vi "Transcriptor LabVIEW to C code Step 3 Translate Elements.vi"(8 "error in (no error)":errorcluster, 11 "Diagram in":refnum<vi>) -> (0 "error out":errorcluster, 1 "transcripted C code":string[](array[string]), 2 "feedback and other output assignments":string[](array[string]), 3 "transcriptor cluster":T1[](array[typedef]))   [LabVIEW 2014]
uses:
  types/LabVIEW Universal Transcriptor Cluster.ctl
  <vilib>/Utility/miscctls.llb/LVPointTypeDef.ctl
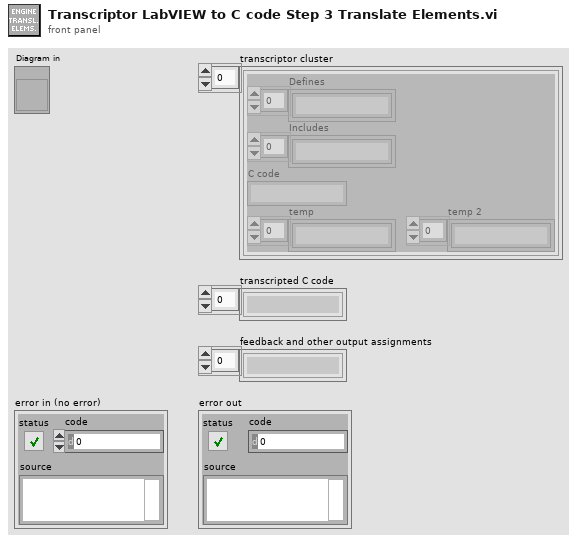
[diagram p1: front panel]
types:
  T1 = typedef "LabVIEW Universal Transcriptor Cluster.ctl" = cluster{"Defines":string[], "Includes":string[], "C code":string, "temp":string[], "temp 2":string[]}
  T2 = typedef "LVPointTypeDef.ctl" = cluster{"Horizontal":i16, "Vertical":i16}
  T3 = cluster{"wire labels":string[], "wire terminals datatypes":string[][]}
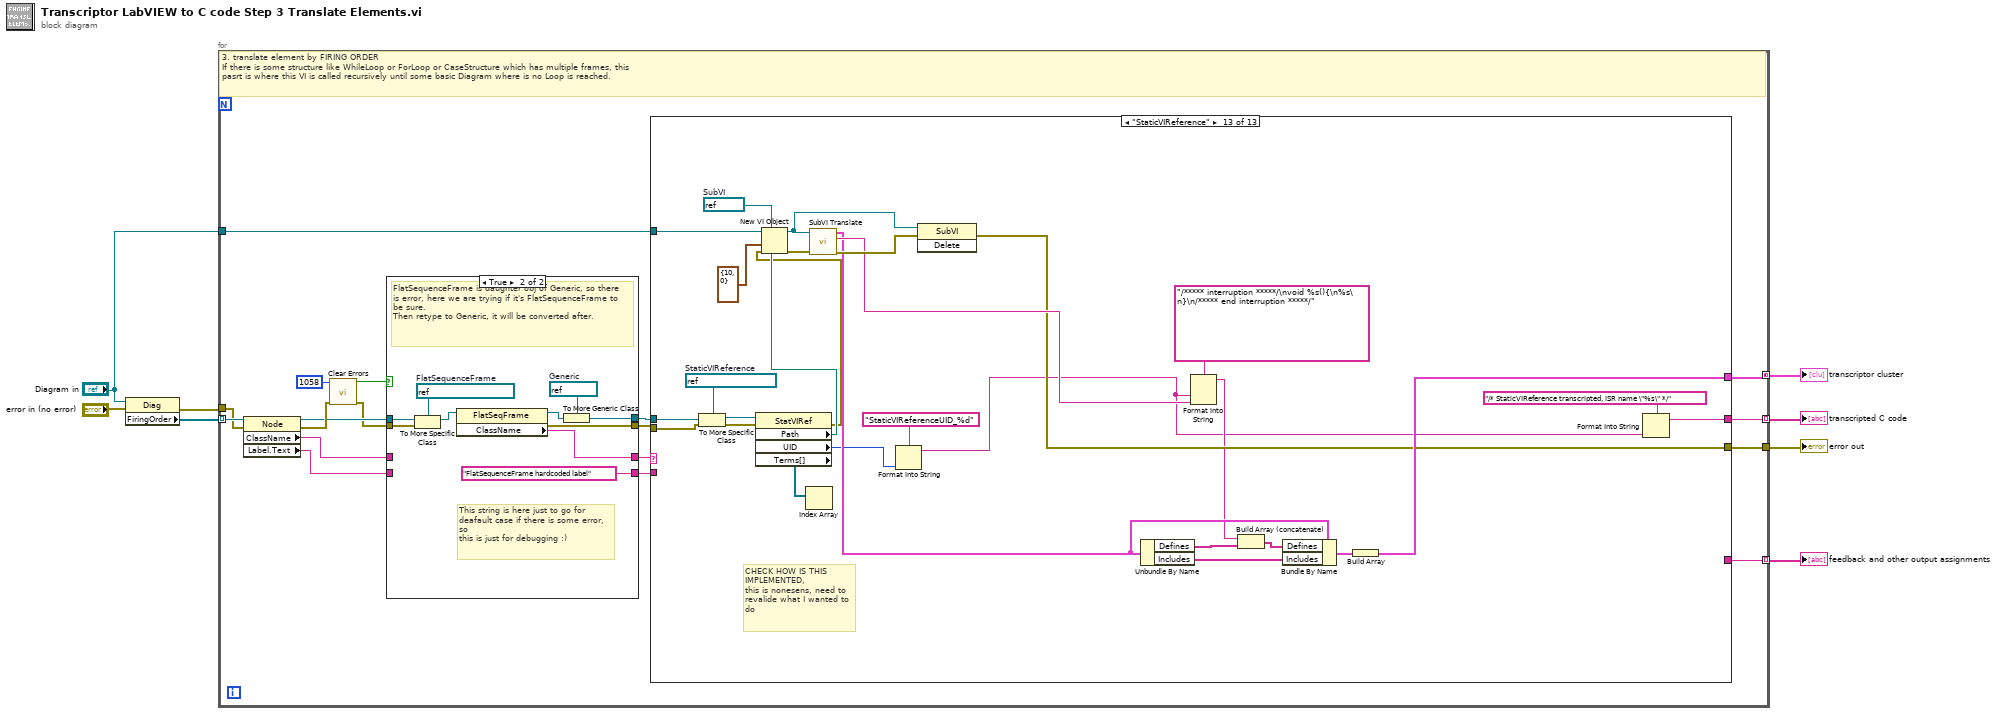
[diagram p0: block diagram]
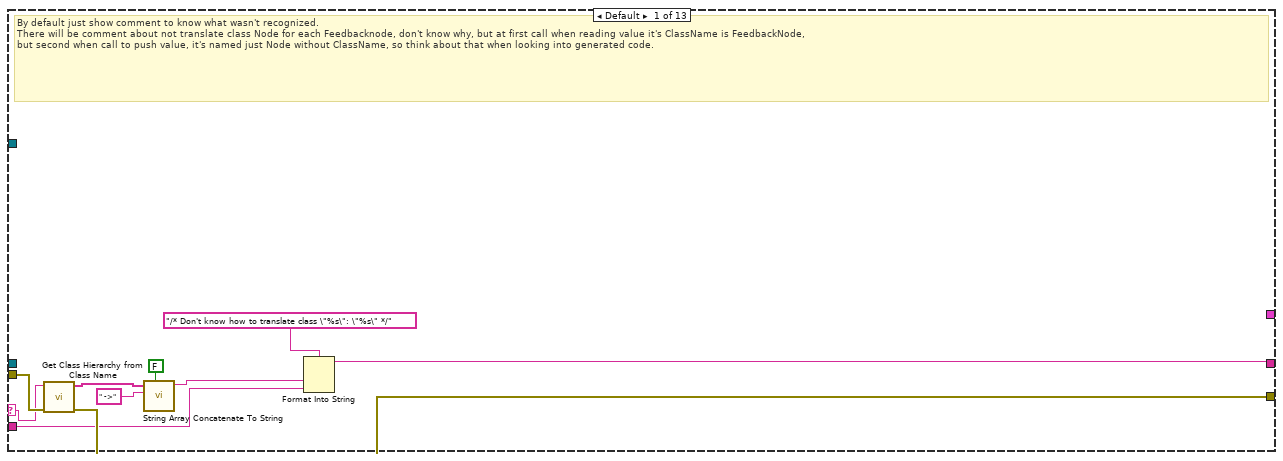
[diagram p3: hidden frame]
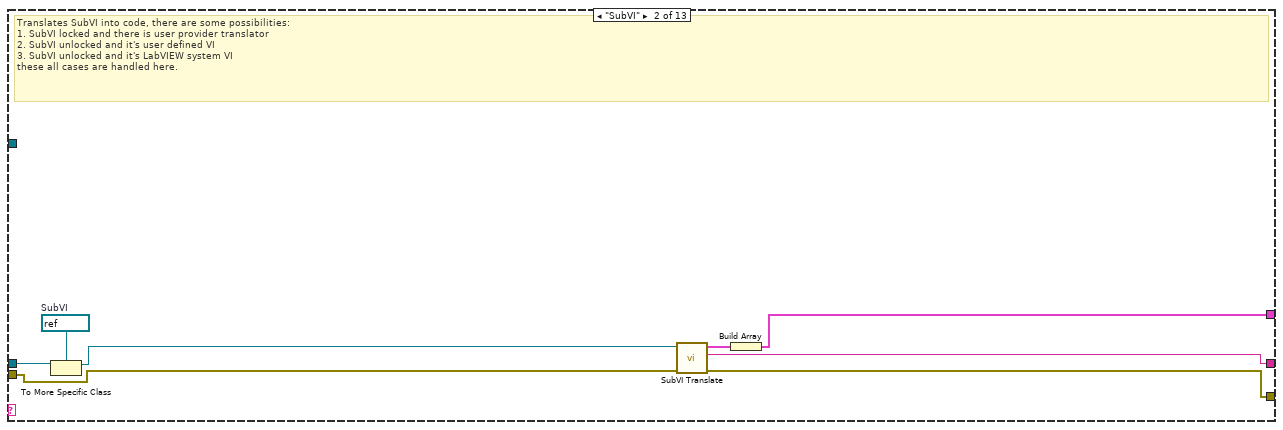
[diagram p4: hidden frame]
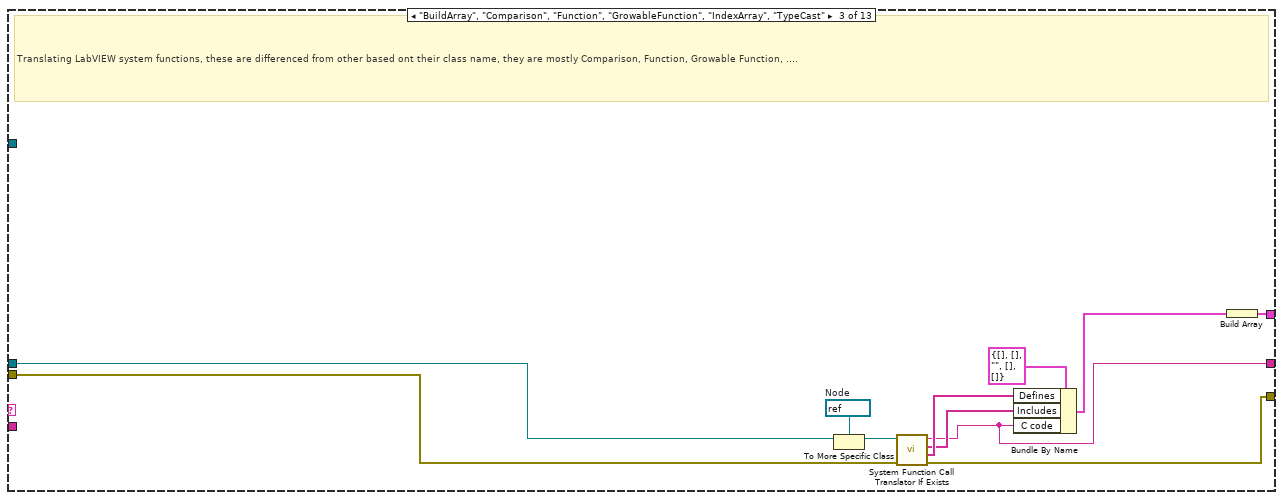
[diagram p5: hidden frame]
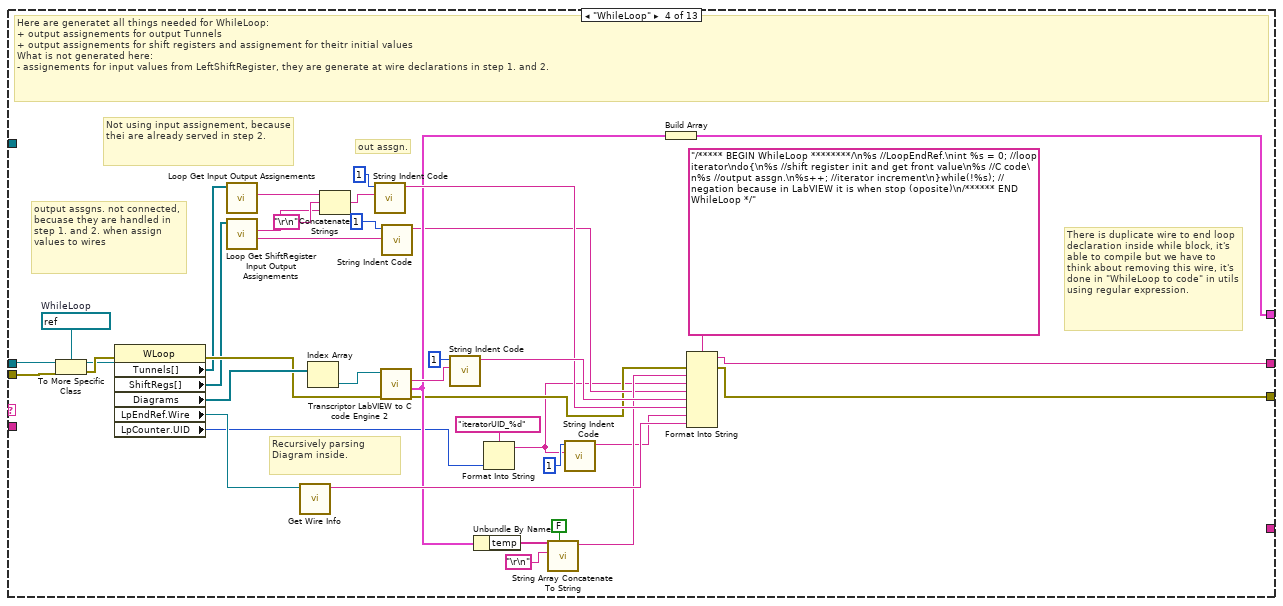
[diagram p6: hidden frame]
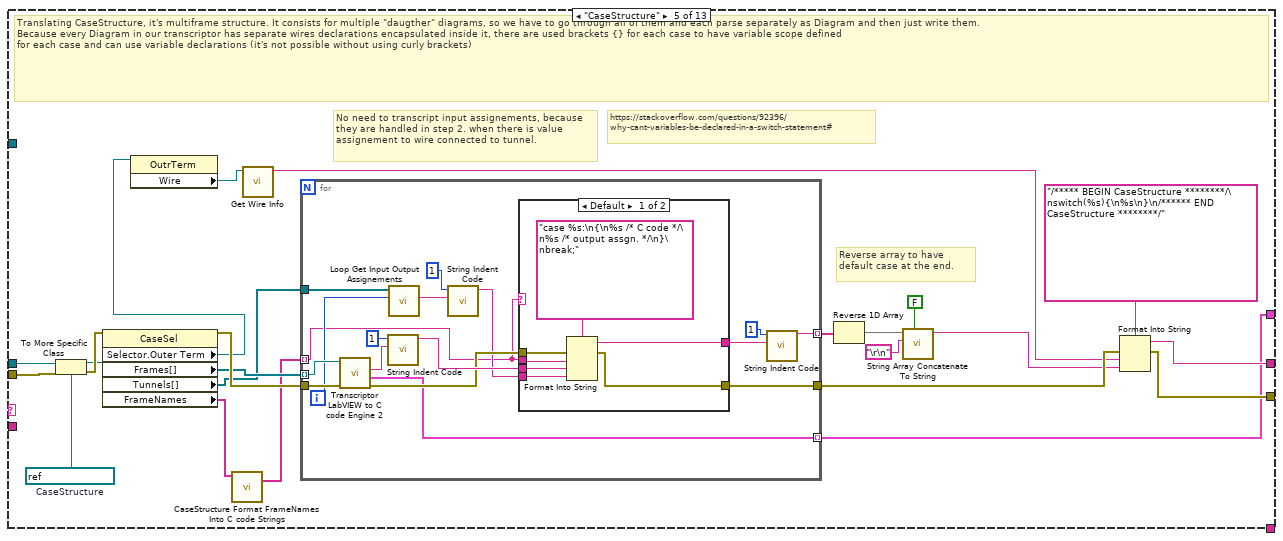
[diagram p7: hidden frame]
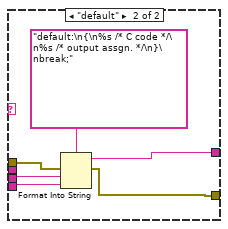
[diagram p8: hidden frame]
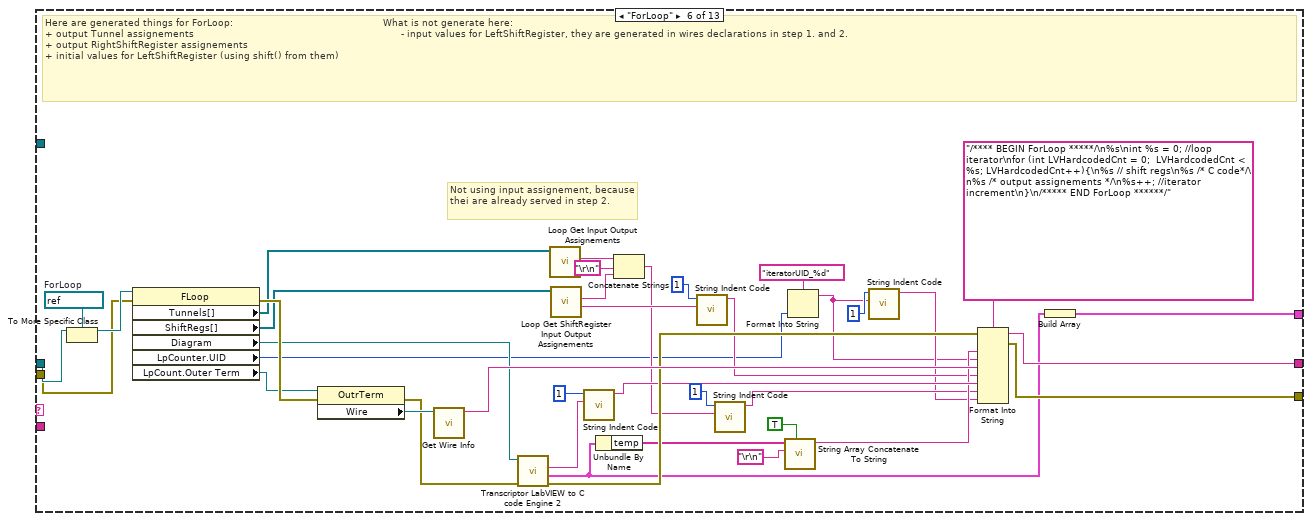
[diagram p9: hidden frame]
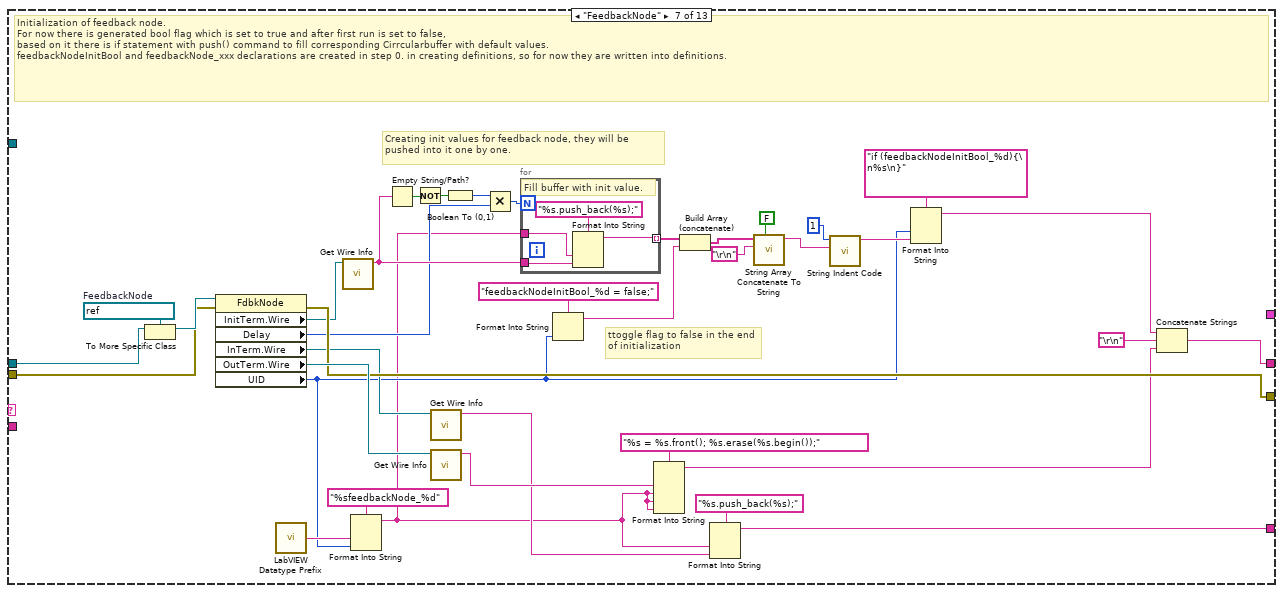
[diagram p10: hidden frame]
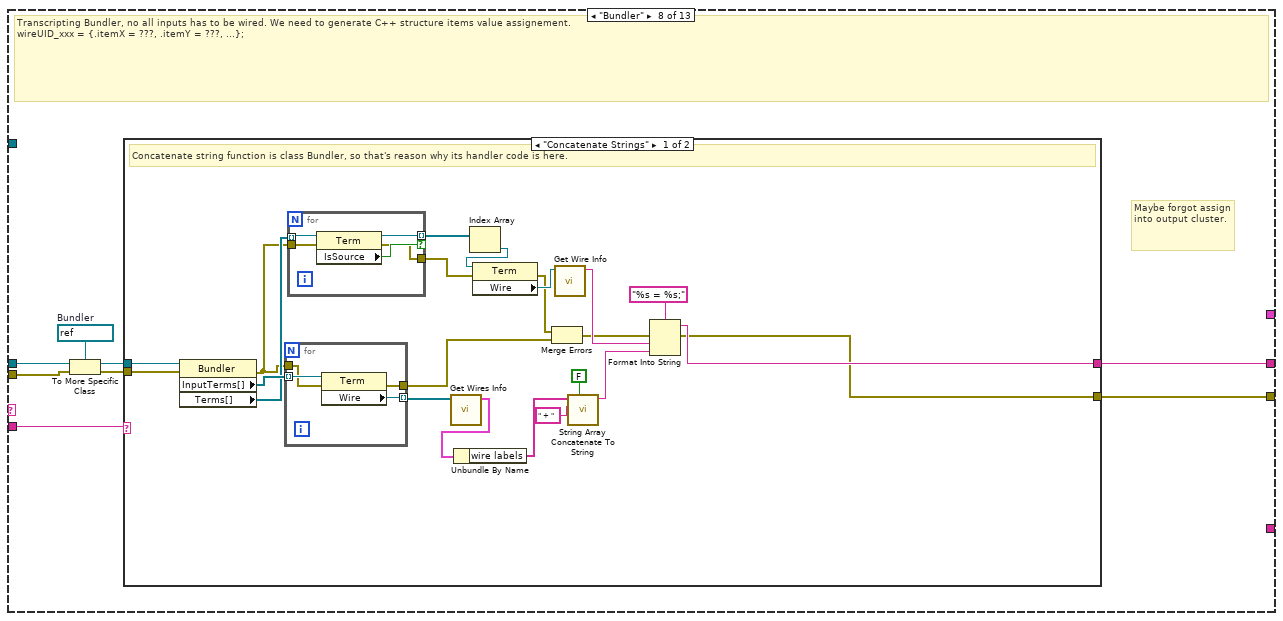
[diagram p11: hidden frame]
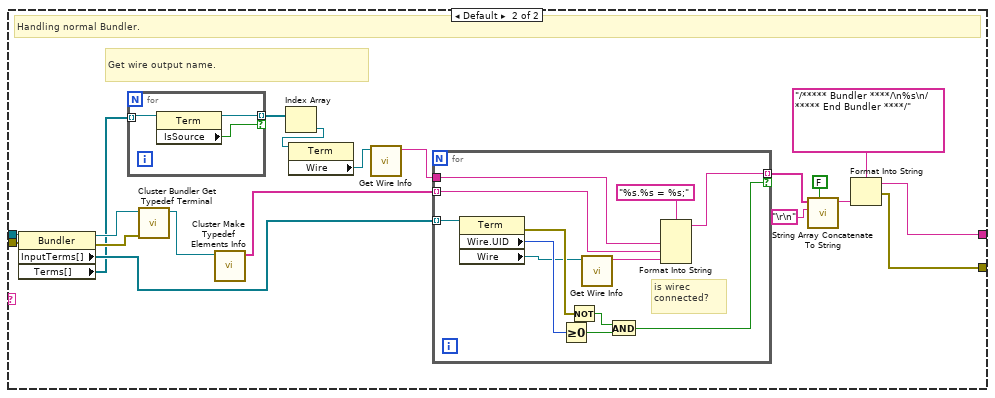
[diagram p12: hidden frame]
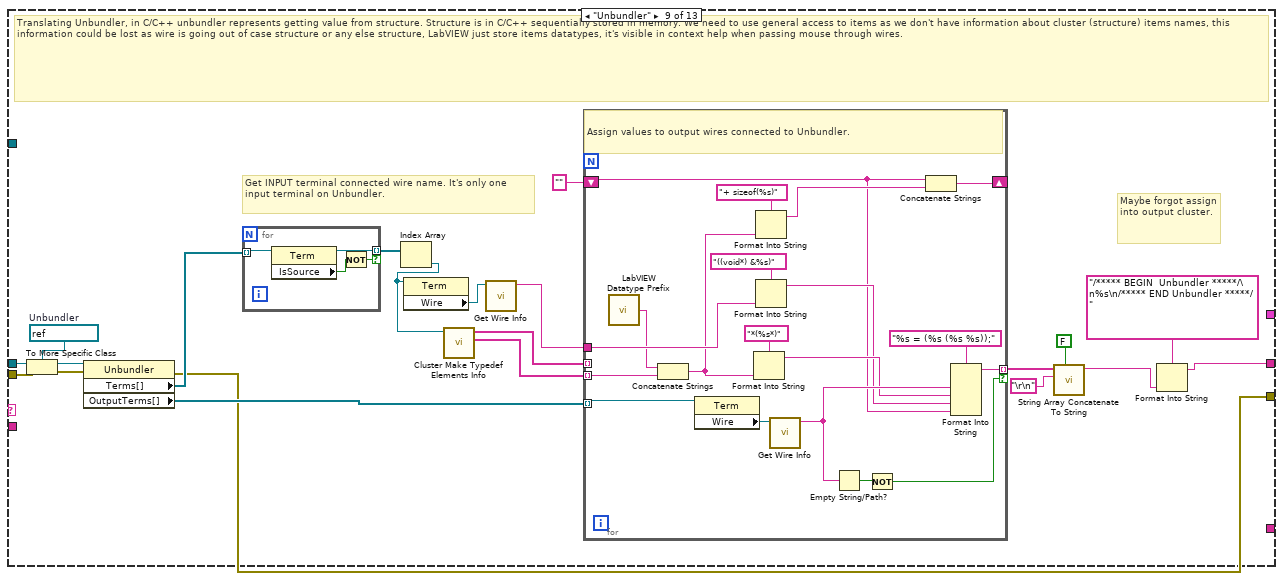
[diagram p13: hidden frame]
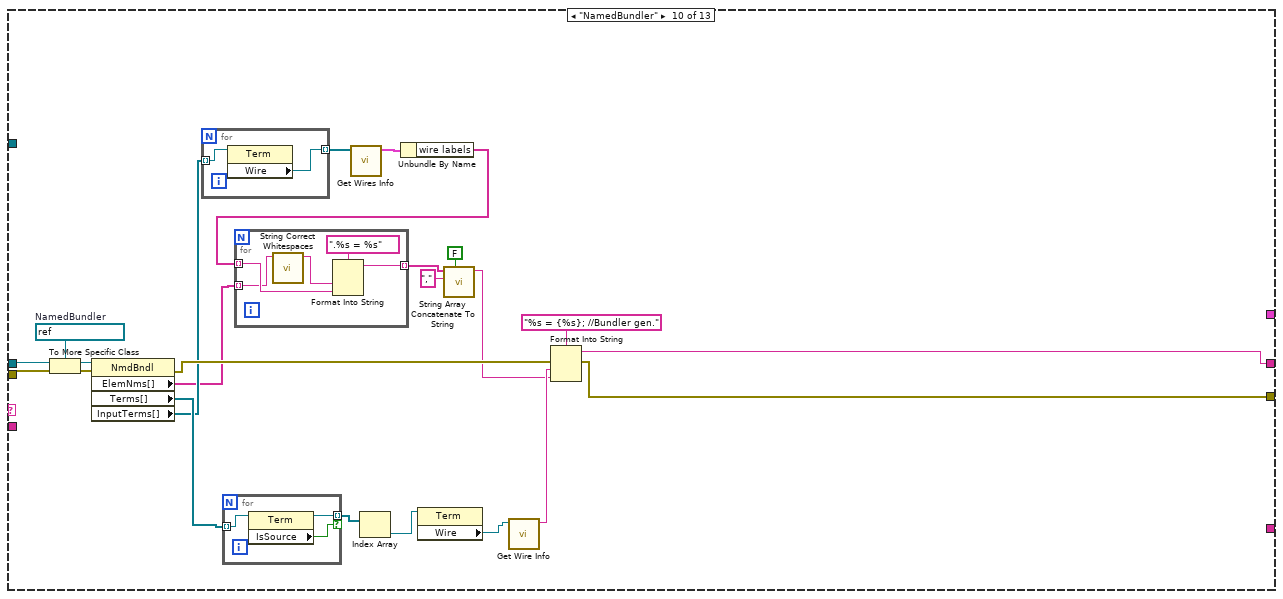
[diagram p14: hidden frame]
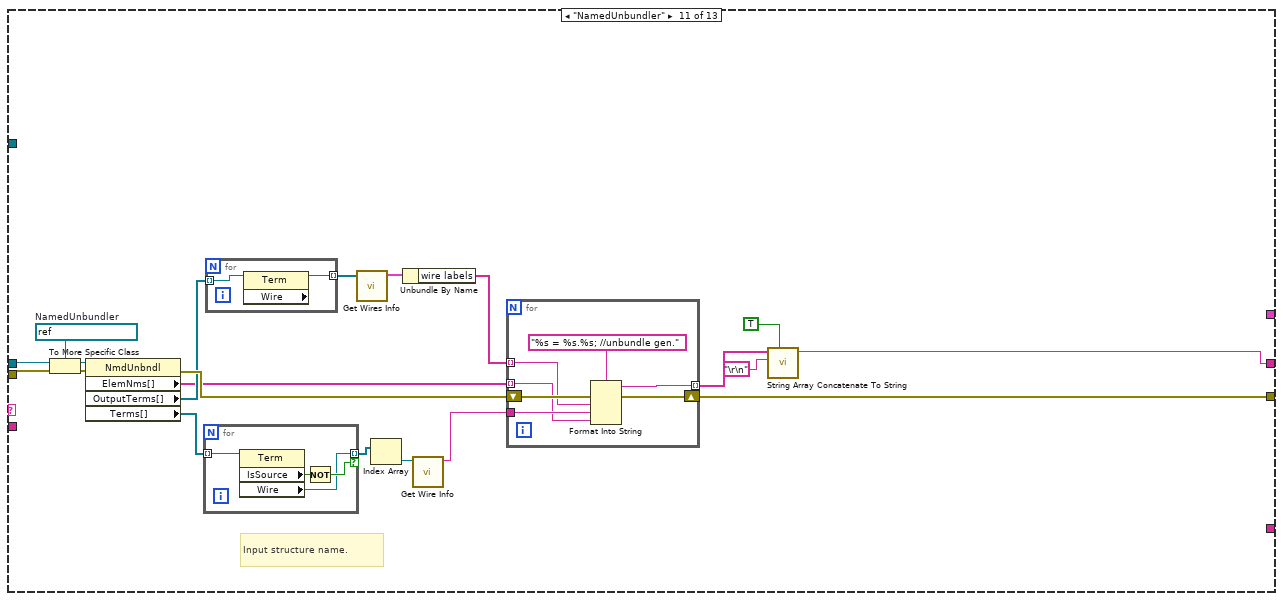
[diagram p15: hidden frame]
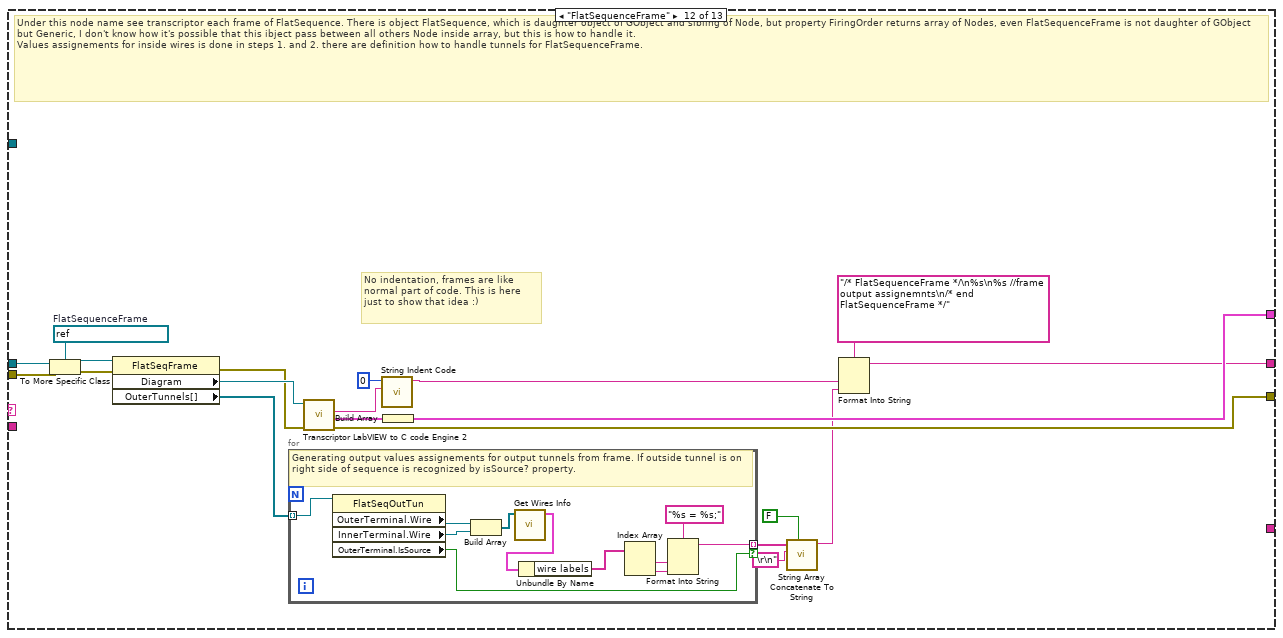
[diagram p16: hidden frame]
diagram:
  n1 = property on="Property Node" class="Diag"(reference="Diagram in", error in="error in (no error)") -> (error out=w3:errorcluster, "FiringOrder"=w8:refnum<vi>[])  [unwired: 1 out]
  n2 = for {
    tunnel: w8 -> [w26] mode=indexing
    tunnel: w3 -> [w25]
    tunnel: [w22] -> w4 mode=indexing
    tunnel: [w21] -> w6
    tunnel: [w24] -> w2 mode=concatenating
    tunnel: [w23] -> w7 mode=indexing
    tunnel: "Diagram in" -> [w9]
    # "3. translate element by FIRING ORDER\nIf there is some structure like WhileLoop or ForLoop or CaseStructure which has multiple frames, this\npasrt is where this VI is called recursively until some basic Diagram where is no Loop is reached."
    n3 = property class="Node"(reference=w26, error in=w25) -> (reference out=w18:refnum<vi>, error out=w20:errorcluster, "ClassName"=w13:string, "Label.Text"=w12:string)
    n4 = call <vilib>:"Clear Errors.vi"("error in (no error)"=w20, "specific error code to clear (0: all)"=1058) -> ("error out"=w17:errorcluster, "specific error cleared?"=w16:bool)  [unwired: 4 in]
    n5 = case shown="True" w16 {
      tunnel: w18 -> [w27 w40]
      tunnel: w17 -> [w28 w39]
      tunnel: [w30 w36] -> w15
      tunnel: [w29 "FlatSequenceFrame hardcoded label" ("Label.Text")] -> w14
      tunnel: w13 -> [w30 _]
      tunnel: w12 -> [w29 _]
      tunnel: [w28 w35] -> w11
      tunnel: [w27 w31] -> w10
      frame False {
        # "No error, so we are parsing some Node."
      }
      frame True {
        w33 = refnum<vi> refnum  # Generic
        w38 = refnum<vi> refnum  # FlatSequenceFrame
        # "This string is here just to go for\ndeafault case if there is some error, so\nthis is just for debugging :)"
        # "FlatSequenceFrame is daughter obj of Generic, so there is error, here we are trying if it's FlatSequenceFrame to be sure.\nThen retype to Generic, it will be converted after."
        n6 = To More Specific Class(target class=w38, reference=w40, error in=w39) -> (specific class reference=w37:refnum<vi>)  [unwired: 1 out]
        n7 = property class="FlatSeqFrame"(reference=w37) -> (reference out=w32:refnum<vi>, error out=w35:errorcluster, "ClassName"=w36:string)  [unwired: 1 in]
        n8 = To More Generic Class(target class=w33, reference=w32) -> (generic class reference=w31:refnum<vi>)
      }
    }
    n9 = case shown="\"StaticVIReference\"" w15 {
      selector: w15 -> [w41 _ _ _ _ _ _ _ _ _ _ _ _]
      tunnel: w10 -> [_ w58 w61 w108 w114 w200 w237 w248 w332 w381 w411 w444 w483]
      tunnel: [w49 w55 w66 w100 w126 w190 w210 w243 w315 w368 w392 w430 w460] -> w22
      tunnel: w11 -> [w44 w54 w69 w104 w129 w197 w229 w247 w331 w380 w410 w440 w482]
      tunnel: [w43 w53 w63 w99 w124 w191 w228 w244 w318 w366 w404 w434 w468] -> w21
      tunnel: [_ w51 w65 w89 w111 w182 _ _ _ _ _ w432 w479] -> w24
      tunnel: w14 -> [w42 _ _ _ _ _ _ w242 _ _ _ _ _]
      tunnel: [_ _ _ _ _ _ w204 _ _ _ _ _ _] -> w23
      tunnel: w9 -> [_ _ _ _ _ _ _ _ _ _ _ _ w477]
      frame Default {
        # "By default just show comment to know what wasn't recognized.\nThere will be comment about not translate class Node for each Feedbacknode, don't know why, but at first call when reading value it's ClassName is FeedbackNode,\nbut second when call to push value, it's named just Node without ClassName, so think about that when looking into generated code."
        n10 = call <vilib>:"Get Class Hierarchy from Class Name.vi"("error in (no error)"=w44, "Class Name"=w41) -> ("error out"=w43:errorcluster, "Class Hierarchy"=w47:string[])  [unwired: 8 in]
        n11 = call "String Array Concatenate To String.vi"("insert last delimiter?"=FALSE, "Delimiter char"=" ->", "Array String In"=w47) -> ("String"=w45:string)  [unwired: 8 in]
        n12 = Format Into String(format string="/* Don't know how to translate class \"%s\": \"%s\" */", w45, w42) -> (resulting string=w49:string)  [unwired: 2 in, 1 out]
      }
      frame "SubVI" {
        w57 = refnum<vi> refnum  # SubVI
        # "Translates SubVI into code, there are some possibilities:\n1. SubVI locked and there is user provider translator\n2. SubVI unlocked and it's user defined VI\n3. SubVI unlocked and it's LabVIEW system VI\nthese all cases are handled here."
        n13 = To More Specific Class(target class=w57, reference=w58) -> (specific class reference=w56:refnum<vi>)  [unwired: 1 in, 1 out]
        n14 = call "SubVI Translate.vi"("error in (no error)"=w54, "SubVI in"=w56) -> ("error out"=w53:errorcluster, "transcripted code"=w55:string, "transcriptor cluster"=w52:T1)  [unwired: 7 in]
        n15 = Build Array(w52) -> (w51:T1[])
      }
      frame "BuildArray", "Comparison", "Function", "GrowableFunction", "IndexArray", "TypeCast" {
        w59 = refnum<vi> refnum  # Node
        # "Translating LabVIEW system functions, these are differenced from other based ont their class name, they are mostly Comparison, Function, Growable Function, ...."
        n16 = To More Specific Class(target class=w59, reference=w61) -> (specific class reference=w60:refnum<vi>)  [unwired: 1 in, 1 out]
        n17 = call "System Function Call Translator If Exists.vi"("Error In"=w69, "Node Refnum"=w60) -> ("Error Out"=w63:errorcluster, "Defines"=w68:string[], "Includes"=w67:string[], "Replaced Code"=w66:string)  [unwired: 6 in]
        n18 = Bundle By Name(cluster=T1 {"Defines"=[], "Includes"=[], "C code"="", "temp"=[], "temp 2"=[]} ("input cluster"), "Defines"=w68, "Includes"=w67, "C code"=w66) -> (w64:T1)
        n19 = Build Array(w64) -> (w65:T1[])
      }
      frame "WhileLoop" {
        w107 = refnum<vi> refnum  # WhileLoop
        # "output assgns. not connected, becuase they are handled in step 1. and 2. when assign values to wires"
        # "Not using input assignement, because thei are already served in step 2."
        # "out assgn."
        # "There is duplicate wire to end loop declaration inside while block, it's able to compile but we have to think about removing this wire, it's done in \"WhileLoop to code\" in utils using regular expression."
        # "Recursively parsing Diagram inside."
        # "Here are generatet all things needed for WhileLoop:\n+ output assignements for output Tunnels\n+ output assignements for shift registers and assignement for theitr initial values\nWhat is not generated here:\n- assignements for input values from LeftShiftRegister, they are generate at wire declarations in step 1. and 2."
        n20 = To More Specific Class(target class=w107, reference=w108, error in=w104) -> (specific class reference=w98:refnum<vi>, error out=w106:errorcluster)
        n21 = property class="WLoop"(reference=w98, error in=w106) -> (error out=w103:errorcluster, "Tunnels[]"=w93:refnum<vi>[], "ShiftRegs[]"=w80:refnum<vi>[], "Diagrams"=w105:refnum<vi>[], "LpEndRef.Wire"=w97:refnum<vi>, "LpCounter.UID"=w73:i32)  [unwired: 1 out]
        n22 = call "Loop Get Input Output Assignements.vi"("Loop Tunnels[]"=w93) -> ("tunnels output assignements"=w84:string)  [unwired: 9 in, 1 out]
        n23 = call "Loop Get ShiftRegister Input Output Assignements.vi"("RightShiftRegister[]"=w80) -> ("init values"=w70:string, "output assignements"=w79:string)  [unwired: 8 in, 1 out]
        n24 = call "Get Wire Info.vi"("Wire"=w97) -> ("wire label"=w92:string)  [unwired: 9 in, 1 out]
        n25 = Index Array(array=w105) -> (element=w102:refnum<vi>)  [unwired: 1 in]
        n26 = Concatenate Strings(w84, "\r\n", w79) -> (w82:string)
        n27 = call "String Indent Code.vi"("complete code"=w82, "actual nested level"=1) -> ("indented code"=w90:string)  [unwired: 9 in]
        n28 = call "Transcriptor LabVIEW to C code Engine 2.vi"("Error In"=w103, "Diagram in"=w102) -> ("error out"=w76:errorcluster, "output cluster"=w88:T1, "transcripted code"=w96:string)  [unwired: 5 in, 2 out]
        n29 = call "String Indent Code.vi"("complete code"=w70, "actual nested level"=1) -> ("indented code"=w77:string)  [unwired: 9 in]
        n30 = call "String Indent Code.vi"("complete code"=w96, "actual nested level"=1) -> ("indented code"=w94:string)  [unwired: 9 in]
        n31 = Unbundle By Name(w88) -> ("temp"=w87:string[])
        n32 = Format Into String(format string="iteratorUID_%d", w73) -> (resulting string=w71:string)  [unwired: 2 in, 1 out]
        n33 = call "String Array Concatenate To String.vi"("insert last delimiter?"=FALSE, "Delimiter char"="\r\n", "Array String In"=w87) -> ("String"=w81:string)  [unwired: 8 in]
        n34 = call "String Indent Code.vi"("complete code"=w71, "actual nested level"=1) -> ("indented code"=w72:string)  [unwired: 9 in]
        n35 = Build Array(w88) -> (w89:T1[])
        n36 = Format Into String(format string="/***** BEGIN WhileLoop ********/\n%s //LoopEndRef.\nint %s = 0; //loop iterator\ndo{\n%s //shift register init and get front value\n%s //C code\n%s //output assgn.\n%s++; //iterator increment\n}while(!%s); //negation because in LabVIEW it is when stop (oposite)\n/****** END WhileLoop */", error in=w76, w81, w71, w77, w94, w90, w72, w92) -> (resulting string=w100:string, error out=w99:errorcluster)  [unwired: 1 in]
      }
      frame "CaseStructure" {
        w131 = refnum<vi> refnum  # CaseStructure
        # "Reverse array to have default case at the end."
        # "https://stackoverflow.com/questions/92396/why-cant-variables-be-declared-in-a-switch-statement#"
        # "No need to transcript input assignements, because they are handled in step 2. when there is value assignement to wire connected to tunnel."
        # "Translating CaseStructure, it's multiframe structure. It consists for multiple \"daugther\" diagrams, so we have to go through all of them and each parse separately as Diagram and then just write them.\nBecause every Diagram in our transcriptor has separate wires declarations encapsulated inside it, there are used brackets {} for each case to have variable scope defined\nfor each case and can use variable declarations (it's not possible without using curly brackets)"
        n37 = To More Specific Class(target class=w131, reference=w114, error in=w129) -> (specific class reference=w123:refnum<vi>, error out=w130:errorcluster)
        n38 = property class="CaseSel"(reference=w123, error in=w130) -> (error out=w128:errorcluster, "Selector.Outer Term"=w121:refnum<vi>, "Frames[]"=w122:refnum<vi>[], "Tunnels[]"=w115:refnum<vi>[], "FrameNames"=w112:string[])  [unwired: 1 out]
        n39 = property class="OutrTerm"(reference=w121) -> ("Wire"=w120:refnum<vi>)  [unwired: 1 in, 2 out]
        n40 = call "CaseStructure Format FrameNames Into C code Strings.vi"("FrameNames in"=w112) -> ("c code cases names"=w113:string[])  [unwired: 10 in]
        n41 = call "Get Wire Info.vi"("Wire"=w120) -> ("wire label"=w119:string)  [unwired: 9 in, 1 out]
        n42 = for {
          tunnel: w128 -> [w148]
          tunnel: [w142] -> w125
          tunnel: w122 -> [w147] mode=indexing
          tunnel: w113 -> [w132] mode=indexing
          tunnel: [w140] -> w110 mode=indexing
          tunnel: w115 -> [w137]
          tunnel: [w133] -> w111 mode=indexing
          i -> [w138]
          n43 = call "Transcriptor LabVIEW to C code Engine 2.vi"("Error In"=w148, "Diagram in"=w147) -> ("error out"=w143:errorcluster, "output cluster"=w133:T1, "transcripted code"=w145:string)  [unwired: 5 in, 2 out]
          n44 = call "String Indent Code.vi"("complete code"=w145, "actual nested level"=1) -> ("indented code"=w144:string)  [unwired: 9 in]
          n45 = call "Loop Get Input Output Assignements.vi"("Inside Terms[] offset"=w138, "Loop Tunnels[]"=w137) -> ("tunnels output assignements"=w135:string)  [unwired: 8 in, 1 out]
          n46 = call "String Indent Code.vi"("complete code"=w135, "actual nested level"=1) -> ("indented code"=w134:string)  [unwired: 9 in]
          n47 = case shown="Default" w132 {
            tunnel: w144 -> [w155 w157]
            tunnel: w132 -> [w154 _]
            tunnel: w143 -> [w152 w156]
            tunnel: [w151 w159] -> w142
            tunnel: [w150 w160] -> w139
            tunnel: w134 -> [w149 w158]
            frame Default {
              n48 = Format Into String(format string="case %s:\n{\n%s /* C code */\n%s /* output assgn. */\n}\nbreak;", error in=w152, w154, w155, w149) -> (resulting string=w150:string, error out=w151:errorcluster)  [unwired: 1 in]
            }
            frame "default" {
              n49 = Format Into String(format string="default:\n{\n%s /* C code */\n%s /* output assgn. */\n}\nbreak;", error in=w156, w157, w158) -> (resulting string=w160:string, error out=w159:errorcluster)  [unwired: 1 in]
            }
          }
          n50 = call "String Indent Code.vi"("complete code"=w139, "actual nested level"=1) -> ("indented code"=w140:string)  [unwired: 9 in]
        }
        n51 = Reverse 1D Array(array=w110) -> (reversed array=w109:string[])
        n52 = call "String Array Concatenate To String.vi"("insert last delimiter?"=FALSE, "Delimiter char"="\r\n", "Array String In"=w109) -> ("String"=w116:string)  [unwired: 8 in]
        n53 = Format Into String(format string="/***** BEGIN CaseStructure ********/\nswitch(%s){\n%s\n}\n/****** END CaseStructure ********/", error in=w125, w119, w116) -> (resulting string=w126:string, error out=w124:errorcluster)  [unwired: 1 in]
      }
      frame "ForLoop" {
        w199 = refnum<vi> refnum  # ForLoop
        # "Not using input assignement, because thei are already served in step 2."
        # "Here are generated things for ForLoop:                                                  What is not generate here:\n+ output Tunnel assignements                                                                     - input values for LeftShiftRegister, they are generated in wires declarations in step 1. and 2.\n+ output RightShiftRegister assignements\n+ initial values for LeftShiftRegister (using shift() from them)"
        n54 = To More Specific Class(target class=w199, reference=w200) -> (specific class reference=w198:refnum<vi>)  [unwired: 1 in, 1 out]
        n55 = property class="FLoop"(reference=w198, error in=w197) -> (error out=w196:errorcluster, "Tunnels[]"=w183:refnum<vi>[], "ShiftRegs[]"=w176:refnum<vi>[], "Diagram"=w189:refnum<vi>, "LpCounter.UID"=w164:i32, "LpCount.Outer Term"=w195:refnum<vi>)  [unwired: 1 out]
        n56 = property class="OutrTerm"(reference=w195, error in=w196) -> (error out=w188:errorcluster, "Wire"=w194:refnum<vi>)  [unwired: 1 out]
        n57 = call "Get Wire Info.vi"("Wire"=w194) -> ("wire label"=w192:string)  [unwired: 9 in, 1 out]
        n58 = call "Transcriptor LabVIEW to C code Engine 2.vi"("Error In"=w188, "Diagram in"=w189) -> ("error out"=w187:errorcluster, "output cluster"=w181:T1, "transcripted code"=w186:string)  [unwired: 5 in, 2 out]
        n59 = call "Loop Get Input Output Assignements.vi"("Loop Tunnels[]"=w183) -> ("tunnels output assignements"=w173:string)  [unwired: 9 in, 1 out]
        n60 = call "Loop Get ShiftRegister Input Output Assignements.vi"("RightShiftRegister[]"=w176) -> ("init values"=w172:string, "output assignements"=w170:string)  [unwired: 8 in, 1 out]
        n61 = call "String Indent Code.vi"("complete code"=w186, "actual nested level"=1) -> ("indented code"=w184:string)  [unwired: 9 in]
        n62 = Unbundle By Name(w181) -> ("temp"=w180:string[])
        n63 = Concatenate Strings(w173, "\r\n", w170) -> (w168:string)
        n64 = call "String Indent Code.vi"("complete code"=w172, "actual nested level"=1) -> ("indented code"=w174:string)  [unwired: 9 in]
        n65 = call "String Indent Code.vi"("complete code"=w168, "actual nested level"=1) -> ("indented code"=w167:string)  [unwired: 9 in]
        n66 = call "String Array Concatenate To String.vi"("insert last delimiter?"=TRUE, "Delimiter char"="\r\n", "Array String In"=w180) -> ("String"=w177:string)  [unwired: 8 in]
        n67 = Format Into String(format string="iteratorUID_%d", w164) -> (resulting string=w162:string)  [unwired: 2 in, 1 out]
        n68 = call "String Indent Code.vi"("complete code"=w162, "actual nested level"=1) -> ("indented code"=w163:string)  [unwired: 9 in]
        n69 = Format Into String(format string="/**** BEGIN ForLoop *****/\n%s\nint %s = 0; //loop iterator\nfor (int LVHardcodedCnt = 0;  LVHardcodedCnt < %s; LVHardcodedCnt++){\n%s // shift regs\n%s /* C code*/\n%s /* output assignements */\n%s++; //iterator increment\n}\n/***** END ForLoop ******/", error in=w187, w177, w162, w192, w174, w184, w167, w163) -> (resulting string=w190:string, error out=w191:errorcluster)  [unwired: 1 in]
        n70 = Build Array(w181) -> (w182:T1[])
      }
      frame "FeedbackNode" {
        w235 = refnum<vi> refnum  # FeedbackNode
        # "Creating init values for feedback node, they will be pushed into it one by one."
        # "ttoggle flag to false in the end of initialization"
        # "Initialization of feedback node.\nFor now there is generated bool flag which is set to true and after first run is set to false,\nbased on it there is if statement with push() command to fill corresponding Cirrcularbuffer with default values.\nfeedbackNodeInitBool and feedbackNode_xxx declarations are created in step 0. in creating definitions, so for now they are written into definitions."
        n71 = To More Specific Class(target class=w235, reference=w237) -> (specific class reference=w236:refnum<vi>)  [unwired: 1 in, 1 out]
        n72 = property class="FdbkNode"(reference=w236, error in=w229) -> (error out=w228:errorcluster, "InitTerm.Wire"=w222:refnum<vi>, "Delay"=w203:i32, "InTerm.Wire"=w223:refnum<vi>, "OutTerm.Wire"=w234:refnum<vi>, "UID"=w214:i32)  [unwired: 1 out]
        n73 = call "LabVIEW Datatype Prefix.vi"() -> ("datatype prefix"=w231:string)
        n74 = call "Get Wire Info.vi"("Wire"=w222) -> ("wire label"=w224:string)  [unwired: 9 in, 1 out]
        n75 = Format Into String(format string="%sfeedbackNode_%d" ("Replaced Code"), w231, w214) -> (resulting string=w201:string)  [unwired: 2 in, 1 out]
        n76 = Empty String/Path?(string/path=w224) -> (empty?=w227:bool)
        n77 = Not(x=w227) -> (.not. x?=w226:bool)
        n78 = call "Get Wire Info.vi"("Wire"=w223) -> ("wire label"=w205:string)  [unwired: 9 in, 1 out]
        n79 = call "Get Wire Info.vi"("Wire"=w234) -> ("wire label"=w230:string)  [unwired: 9 in, 1 out]
        n80 = Boolean To (0,1)(Boolean=w226) -> (0, 1=w202:i16)
        n81 = Multiply(x=w202, y=w203) -> (x*y=w225:i32)
        n82 = for {
          N: w225 -> [_]
          tunnel: [w240] -> w213 mode=indexing
          tunnel: w201 -> [w239]
          tunnel: w224 -> [w238]
          # "Fill buffer with init value."
          n83 = Format Into String(format string="%s.push_back(%s);", w239, w238) -> (resulting string=w240:string)  [unwired: 2 in, 1 out]
        }
        n84 = Format Into String(format string="feedbackNodeInitBool_%d = false;", w214) -> (resulting string=w212:string)  [unwired: 2 in, 1 out]
        n85 = Format Into String(format string="%s = %s.front(); %s.erase(%s.begin());" ("Replaced Code"), w230, w201, w201, w201) -> (resulting string=w208:string)  [unwired: 2 in, 1 out]
        n86 = Build Array (concatenate)(w213, w212) -> (w211:string[])
        n87 = Format Into String(format string="%s.push_back(%s);" ("Replaced Code"), w201, w205) -> (resulting string=w204:string)  [unwired: 2 in, 1 out]
        n88 = call "String Array Concatenate To String.vi"("insert last delimiter?"=FALSE, "Delimiter char"="\r\n", "Array String In"=w211) -> ("String"=w218:string)  [unwired: 8 in]
        n89 = call "String Indent Code.vi"("complete code"=w218, "actual nested level"=1) -> ("indented code"=w216:string)  [unwired: 9 in]
        n90 = Format Into String(format string="if (feedbackNodeInitBool_%d){\n%s\n}", w214, w216) -> (resulting string=w209:string)  [unwired: 2 in, 1 out]
        n91 = Concatenate Strings(w209, "\r\n", w208) -> (w210:string)
      }
      frame "Bundler" {
        w249 = refnum<vi> refnum  # Bundler
        # "Maybe forgot assign into output cluster."
        # "Transcripting Bundler, no all inputs has to be wired. We need to generate C++ structure items value assignement.\nwireUID_xxx = {.itemX = ???, .itemY = ???, ...};"
        n92 = To More Specific Class(target class=w249, reference=w248, error in=w247) -> (specific class reference=w246:refnum<vi>, error out=w245:errorcluster)
        n93 = case shown="\"Concatenate Strings\"" w242 {
          tunnel: w246 -> [w271 w299]
          tunnel: w245 -> [w270 w298]
          tunnel: [w252 w290] -> w244
          tunnel: [w256 w289] -> w243
          frame "Concatenate Strings" {
            # "Concatenate string function is class Bundler, so that's reason why its handler code is here."
            n94 = property class="Bundler"(reference=w271, error in=w270) -> (error out=w255:errorcluster, "InputTerms[]"=w269:refnum<vi>[], "Terms[]"=w260:refnum<vi>[])  [unwired: 1 out]
            n95 = for {
              tunnel: w269 -> [w280] mode=indexing
              tunnel: [w279] -> w268 mode=indexing
              tunnel: w255 -> [w278]
              tunnel: [w277] -> w254
              n96 = property class="Term"(reference=w280, error in=w278) -> (error out=w277:errorcluster, "Wire"=w279:refnum<vi>)  [unwired: 1 out]
            }
            n97 = for {
              tunnel: w260 -> [w276] mode=indexing
              tunnel: [w275] -> w263 mode=indexing if=w274
              tunnel: w255 -> [w273]
              tunnel: [w272] -> w251
              n98 = property class="Term"(reference=w276, error in=w273) -> (reference out=w275:refnum<vi>, error out=w272:errorcluster, "IsSource"=w274:bool)
            }
            n99 = call "Get Wires Info.vi"("connected\nwires refs."=w268) -> ("wires info cluster"=w267:T3)  [unwired: 10 in]
            n100 = Unbundle By Name(w267) -> ("wire labels"=w266:string[])
            n101 = Index Array(array=w263) -> (element=w262:refnum<vi>)  [unwired: 1 in]
            n102 = property class="Term"(reference=w262, error in=w251) -> (error out=w250:errorcluster, "Wire"=w261:refnum<vi>)  [unwired: 1 out]
            n103 = Merge Errors(w250, w254) -> (w253:errorcluster)
            n104 = call "Get Wire Info.vi"("Wire"=w261) -> ("wire label"=w258:string)  [unwired: 9 in, 1 out]
            n105 = call "String Array Concatenate To String.vi"("insert last delimiter?"=FALSE, "Delimiter char"=" + ", "Array String In"=w266) -> ("String"=w257:string)  [unwired: 8 in]
            n106 = Format Into String(format string="%s = %s;", error in=w253, w258, w257) -> (resulting string=w256:string, error out=w252:errorcluster)  [unwired: 1 in]
          }
          frame Default {
            # "Get wire output name."
            # "Handling normal Bundler."
            n107 = property class="Bundler"(reference=w299, error in=w298) -> (reference out=w297:refnum<vi>, error out=w296:errorcluster, "InputTerms[]"=w294:refnum<vi>[], "Terms[]"=w288:refnum<vi>[])
            n108 = for {
              tunnel: w288 -> [w302] mode=indexing
              tunnel: [w301] -> w287 mode=indexing if=w300
              n109 = property class="Term"(reference=w302) -> (reference out=w301:refnum<vi>, "IsSource"=w300:bool)  [unwired: 1 in, 1 out]
            }
            n110 = call "Cluster Bundler Get Typedef Terminal.vi"("error in (no error)"=w296, "GObject in"=w297) -> ("Terminal out"=w284:refnum<vi>)  [unwired: 8 in, 1 out]
            n111 = call "Cluster Make Typedef Elements Info.vi"("Terminal in"=w284) -> ("Cluster elements names"=w283:string[])  [unwired: 6 in, 4 out]
            n112 = Index Array(array=w287) -> (element=w286:refnum<vi>)  [unwired: 1 in]
            n113 = property class="Term"(reference=w286) -> ("Wire"=w285:refnum<vi>)  [unwired: 1 in, 2 out]
            n114 = call "Get Wire Info.vi"("Wire"=w285) -> ("wire label"=w282:string)  [unwired: 9 in, 1 out]
            n115 = for {
              tunnel: w294 -> [w314] mode=indexing
              tunnel: w283 -> [w306] mode=indexing
              tunnel: [w304] -> w293 mode=indexing if=w309
              tunnel: w282 -> [w303]
              # "is wirec connected?"
              n116 = property class="Term"(reference=w314) -> (error out=w311:errorcluster, "Wire.UID"=w313:i32, "Wire"=w308:refnum<vi>)  [unwired: 1 in, 1 out]
              n117 = Greater Or Equal To 0?(x=w313) -> (x >= 0?=w312:bool)
              n118 = Not(x=w311) -> (.not. x?=w310:bool)
              n119 = call "Get Wire Info.vi"("Wire"=w308) -> ("wire label"=w305:string)  [unwired: 9 in, 1 out]
              n120 = And(x=w310, y=w312) -> (x .and. y?=w309:bool)
              n121 = Format Into String(format string="%s.%s = %s;", w303, w306, w305) -> (resulting string=w304:string)  [unwired: 2 in, 1 out]
            }
            n122 = call "String Array Concatenate To String.vi"("insert last delimiter?"=FALSE, "Delimiter char"="\r\n", "Array String In"=w293) -> ("String"=w291:string)  [unwired: 8 in]
            n123 = Format Into String(format string="/***** Bundler ****/\n%s\n/***** End Bundler ****/", w291) -> (resulting string=w289:string, error out=w290:errorcluster)  [unwired: 2 in]
          }
        }
      }
      frame "Unbundler" {
        w335 = refnum<vi> refnum  # Unbundler
        # "Maybe forgot assign into output cluster."
        # "Get INPUT terminal connected wire name. It's only one input terminal on Unbundler."
        # "Translating Unbundler, in C/C++ unbundler represents getting value from structure. Structure is in C/C++ sequentially stored in memory. We need to use general access to items as we don't have information about cluster (structure) items names, this information could be lost as wire is going out of case structure or any else structure, LabVIEW just store items datatypes, it's visible in context help when passing mouse through wires."
        n124 = To More Specific Class(target class=w335, reference=w332, error in=w331) -> (specific class reference=w334:refnum<vi>, error out=w333:errorcluster)
        n125 = property class="Unbundler"(reference=w334, error in=w333) -> (error out=w318:errorcluster, "Terms[]"=w328:refnum<vi>[], "OutputTerms[]"=w326:refnum<vi>[])  [unwired: 1 out]
        n126 = for {
          tunnel: w328 -> [w358] mode=indexing
          tunnel: [w357] -> w330 mode=indexing if=w355
          n127 = property class="Term"(reference=w358) -> (reference out=w357:refnum<vi>, "IsSource"=w356:bool)  [unwired: 1 in, 1 out]
          n128 = Not(x=w356) -> (.not. x?=w355:bool)
        }
        n129 = Index Array(array=w330) -> (element=w325:refnum<vi>)  [unwired: 1 in]
        n130 = property class="Term"(reference=w325) -> ("Wire"=w329:refnum<vi>)  [unwired: 1 in, 2 out]
        n131 = call "Cluster Make Typedef Elements Info.vi"("Terminal in"=w325) -> ("Cluster elements datatypes"=w320:string[], "Cluster elements names"=w324:string[])  [unwired: 6 in, 3 out]
        n132 = call "Get Wire Info.vi"("Wire"=w329) -> ("wire label"=w327:string)  [unwired: 9 in, 1 out]
        n133 = for {
          tunnel: w327 -> [w348]
          tunnel: w326 -> [w353] mode=indexing
          tunnel: w324 -> [_] mode=indexing
          tunnel: [w352] -> w323 mode=indexing if=w342
          tunnel: w320 -> [w345] mode=indexing
          shift-right: [w351] -> _
          shift-left: "" ("format string") -> [w338]
          # "Assign values to output wires connected to Unbundler."
          n134 = call "LabVIEW Datatype Prefix.vi"() -> ("datatype prefix"=w336:string)
          n135 = Concatenate Strings(w336, w345) -> (w337:string)
          n136 = property class="Term"(reference=w353) -> ("Wire"=w344:refnum<vi>)  [unwired: 1 in, 2 out]
          n137 = Format Into String(format string="*(%s*)", w337) -> (resulting string=w340:string)  [unwired: 2 in, 1 out]
          n138 = Format Into String(format string="+ sizeof(%s)", w337) -> (resulting string=w349:string)  [unwired: 2 in, 1 out]
          n139 = Format Into String(format string="((void*) &%s)", w348) -> (resulting string=w339:string)  [unwired: 2 in, 1 out]
          n140 = call "Get Wire Info.vi"("Wire"=w344) -> ("wire label"=w341:string)  [unwired: 9 in, 1 out]
          n141 = Empty String/Path?(string/path=w341) -> (empty?=w343:bool)
          n142 = Not(x=w343) -> (.not. x?=w342:bool)
          n143 = Concatenate Strings(w338, w349) -> (w351:string)
          n144 = Format Into String(format string="%s = (%s (%s %s));", w341, w340, w339, w338) -> (resulting string=w352:string)  [unwired: 2 in, 1 out]
        }
        n145 = call "String Array Concatenate To String.vi"("insert last delimiter?"=FALSE, "Delimiter char"="\r\n", "Array String In"=w323) -> ("String"=w316:string)  [unwired: 8 in]
        n146 = Format Into String(format string="/***** BEGIN  Unbundler *****/\n%s\n/***** END Unbundler *****/", w316) -> (resulting string=w315:string)  [unwired: 2 in, 1 out]
      }
      frame "NamedBundler" {
        w378 = refnum<vi> refnum  # NamedBundler
        n147 = To More Specific Class(target class=w378, reference=w381, error in=w380) -> (specific class reference=w377:refnum<vi>, error out=w379:errorcluster)
        n148 = property class="NmdBndl"(reference=w377, error in=w379) -> (error out=w367:errorcluster, "ElemNms[]"=w363:string[], "Terms[]"=w373:refnum<vi>[], "InputTerms[]"=w365:refnum<vi>[])  [unwired: 1 out]
        n149 = for {
          tunnel: w365 -> [w388] mode=indexing
          tunnel: [w387] -> w364 mode=indexing
          n150 = property class="Term"(reference=w388) -> ("Wire"=w387:refnum<vi>)  [unwired: 1 in, 2 out]
        }
        n151 = for {
          tunnel: w373 -> [w391] mode=indexing
          tunnel: [w390] -> w372 mode=indexing if=w389
          n152 = property class="Term"(reference=w391) -> (reference out=w390:refnum<vi>, "IsSource"=w389:bool)  [unwired: 1 in, 1 out]
        }
        n153 = call "Get Wires Info.vi"("connected\nwires refs."=w364) -> ("wires info cluster"=w362:T3)  [unwired: 10 in]
        n154 = Index Array(array=w372) -> (element=w371:refnum<vi>)  [unwired: 1 in]
        n155 = Unbundle By Name(w362) -> ("wire labels"=w361:string[])
        n156 = for {
          tunnel: w363 -> [w383] mode=indexing
          tunnel: w361 -> [w385] mode=indexing
          tunnel: [w384] -> w360 mode=indexing
          n157 = call "String Correct Whitespaces.vi"("String in"=w383) -> ("String out"=w382:string)  [unwired: 10 in]
          n158 = Format Into String(format string=".%s = %s" ("Delimiter char"), w382, w385) -> (resulting string=w384:string)  [unwired: 2 in, 1 out]
        }
        n159 = property class="Term"(reference=w371) -> ("Wire"=w370:refnum<vi>)  [unwired: 1 in, 2 out]
        n160 = call "String Array Concatenate To String.vi"("insert last delimiter?"=FALSE, "Delimiter char"=",", "Array String In"=w360) -> ("String"=w359:string)  [unwired: 8 in]
        n161 = call "Get Wire Info.vi"("Wire"=w370) -> ("wire label"=w369:string)  [unwired: 9 in, 1 out]
        n162 = Format Into String(format string="%s = {%s}; //Bundler gen." ("Delimiter char"), error in=w367, w369, w359) -> (resulting string=w368:string, error out=w366:errorcluster)  [unwired: 1 in]
      }
      frame "NamedUnbundler" {
        w408 = refnum<vi> refnum  # NamedUnbundler
        # "Input structure name."
        n163 = To More Specific Class(target class=w408, reference=w411, error in=w410) -> (specific class reference=w407:refnum<vi>, error out=w409:errorcluster)
        n164 = property class="NmdUnbndl"(reference=w407, error in=w409) -> (error out=w405:errorcluster, "ElemNms[]"=w398:string[], "OutputTerms[]"=w400:refnum<vi>[], "Terms[]"=w403:refnum<vi>[])  [unwired: 1 out]
        n165 = for {
          tunnel: w403 -> [w424] mode=indexing
          tunnel: [w421] -> w402 mode=indexing if=w422
          n166 = property class="Term"(reference=w424) -> ("IsSource"=w423:bool, "Wire"=w421:refnum<vi>)  [unwired: 1 in, 2 out]
          n167 = Not(x=w423) -> (.not. x?=w422:bool)
        }
        n168 = for {
          tunnel: w400 -> [w420] mode=indexing
          tunnel: [w419] -> w399 mode=indexing
          n169 = property class="Term"(reference=w420) -> ("Wire"=w419:refnum<vi>)  [unwired: 1 in, 2 out]
        }
        n170 = call "Get Wires Info.vi"("connected\nwires refs."=w399) -> ("wires info cluster"=w397:T3)  [unwired: 10 in]
        n171 = Index Array(array=w402) -> (element=w401:refnum<vi>)  [unwired: 1 in]
        n172 = Unbundle By Name(w397) -> ("wire labels"=w396:string[])
        n173 = call "Get Wire Info.vi"("Wire"=w401) -> ("wire label"=w406:string)  [unwired: 9 in, 1 out]
        n174 = for {
          shift-right: [w415] -> w404
          shift-left: w405 -> [w416]
          tunnel: w406 -> [w414]
          tunnel: [w417] -> w395 mode=indexing
          tunnel: w398 -> [w413] mode=indexing
          tunnel: w396 -> [w412] mode=indexing
          n175 = Format Into String(format string="%s = %s.%s; //unbundle gen." ("Delimiter char"), error in=w416, w412, w414, w413) -> (resulting string=w417:string, error out=w415:errorcluster)  [unwired: 1 in]
        }
        n176 = call "String Array Concatenate To String.vi"("insert last delimiter?"=TRUE, "Delimiter char"="\r\n", "Array String In"=w395) -> ("String"=w392:string)  [unwired: 8 in]
      }
      frame "FlatSequenceFrame" {
        w443 = refnum<vi> refnum  # FlatSequenceFrame
        # "No indentation, frames are like normal part of code. This is here just to show that idea :)"
        # "Under this node name see transcriptor each frame of FlatSequence. There is object FlatSequence, which is daughter object of GObject and sibling of Node, but property FiringOrder returns array of Nodes, even FlatSequenceFrame is not daughter of GObject but Generic, I don't know how it's possible that this ibject pass between all others Node inside array, but this is how to handle it.\nValues assignements for inside wires is done in steps 1. and 2. there are definition how to handle tunnels for FlatSequenceFrame."
        n177 = To More Specific Class(target class=w443, reference=w444, error in=w440) -> (specific class reference=w442:refnum<vi>, error out=w439:errorcluster)
        n178 = property on="Property Node" class="FlatSeqFrame"(reference=w442, error in=w439) -> (error out=w435:errorcluster, "Diagram"=w441:refnum<vi>, "OuterTunnels[]"=w429:refnum<vi>[])  [unwired: 1 out]
        n179 = for {
          tunnel: w429 -> [w455] mode=indexing
          tunnel: [w446] -> w428 mode=indexing if=w445
          # "Generating output values assignements for output tunnels from frame. If outside tunnel is on right side of sequence is recognized by isSource? property."
          n180 = property on="Property Node" class="FlatSeqOutTun"(reference=w455) -> ("OuterTerminal.Wire"=w454:refnum<vi>, "InnerTerminal.Wire"=w453:refnum<vi>, "OuterTerminal.IsSource"=w445:bool)  [unwired: 1 in, 2 out]
          n181 = Build Array(w454, w453) -> (w452:refnum<vi>[])
          n182 = call "Get Wires Info.vi"("connected\nwires refs."=w452) -> ("wires info cluster"=w451:T3)  [unwired: 10 in]
          n183 = Unbundle By Name(w451) -> ("wire labels"=w450:string[])
          n184 = Index Array(array=w450) -> (element #1=w448:string, element #2=w447:string)  [unwired: 2 in]
          n185 = Format Into String(format string="%s = %s;", w448, w447) -> (resulting string=w446:string)  [unwired: 2 in, 1 out]
        }
        n186 = call "Transcriptor LabVIEW to C code Engine 2.vi"("Error In"=w435, "Diagram in"=w441) -> ("error out"=w434:errorcluster, "output cluster"=w433:T1, "transcripted code"=w438:string)  [unwired: 5 in, 2 out]
        n187 = call "String Indent Code.vi"("complete code"=w438, "actual nested level"=0) -> ("indented code"=w431:string)  [unwired: 9 in]
        n188 = Build Array(w433) -> (w432:T1[])
        n189 = call "String Array Concatenate To String.vi"("insert last delimiter?"=FALSE, "Delimiter char"="\r\n", "Array String In"=w428) -> ("String"=w425:string)  [unwired: 8 in]
        n190 = Format Into String(format string="/* FlatSequenceFrame */\n%s\n%s //frame output assignemnts\n/* end FlatSequenceFrame */", w431, w425) -> (resulting string=w430:string)  [unwired: 2 in, 1 out]
      }
      frame "StaticVIReference" {
        w476 = refnum<vi> refnum  # SubVI
        w484 = refnum<vi> refnum  # StaticVIReference
        # "CHECK HOW IS THIS IMPLEMENTED,\nthis is nonesens, need to revalide what I wanted to do"
        n191 = To More Specific Class(target class=w484, reference=w483, error in=w482) -> (specific class reference=w478:refnum<vi>, error out=w481:errorcluster)
        n192 = property class="StatVIRef"(reference=w478, error in=w481) -> (error out=w469:errorcluster, "Path"=w475:path, "UID"=w458:i32, "Terms[]"=w456:refnum<vi>[])  [unwired: 1 out]
        n193 = New VI Object(vi object class=w476, owner refnum=w477, position/next to=T2 {"Horizontal"=10, "Vertical"=0} ("location"), 6:w475, 8:w469) -> (object refnum=w472:refnum<vi>, 0:w473:errorcluster)  [unwired: 3 in]
        n194 = Index Array(array=w456) -> ()  [unwired: 1 in, 1 out]
        n195 = call "SubVI Translate.vi"("error in (no error)"=w473, "SubVI in"=w472) -> ("error out"=w474:errorcluster, "transcripted code"=w470:string, "transcriptor cluster"=w466:T1)  [unwired: 7 in]
        n196 = Format Into String(format string="StaticVIReferenceUID_%d", w458) -> (resulting string=w457:string)  [unwired: 2 in, 1 out]
        n197 = invoke class="SubVI" method="Delete"(reference=w472, error in=w474) -> (error out=w468:errorcluster)  [unwired: 1 in, 2 out]
        n198 = Unbundle By Name(w466) -> ("Defines"=w463:string[], "Includes"=w465:string[])
        n199 = Format Into String(format string="/***** interruption *****/\nvoid %s(){\n%s\n}\n/***** end interruption *****/", w457, w470) -> (resulting string=w462:string)  [unwired: 2 in, 1 out]
        n200 = Build Array (concatenate)(w462, w463) -> (w464:string[])
        n201 = Bundle By Name(cluster=w466, "Defines"=w464, "Includes"=w465) -> (w467:T1)
        n202 = Build Array(w467) -> (w479:T1[])
        n203 = Format Into String(format string="/* StaticVIReference transcripted, ISR name \"%s\" */", w457) -> (resulting string=w460:string)  [unwired: 2 in, 1 out]
      }
    }
  }
  "feedback and other output assignments" <- w7
  "error out" <- w6
  "transcriptor cluster" <- w2
  "transcripted C code" <- w4
